vi "Get Device Parameters.vi"(8 "error in":errorcluster, 11 "custom device ref":T2=18446744073709551615 format="%.0x") -> (0 "error out":errorcluster, 2 "device parameters":T1, 3 "custom device ref out":T2 format="%.0x")   [LabVIEW 2020, in "AIM ARINC 429 Scripting.lvlib"]
doc: "Returns AIM hardware device parameters such as <b>pxi slot</b>."
uses:
  AIM ARINC 429 Scripting.lvlib
  <vilib>/NI VeriStand/Custom Device API/Custom Device Item Ref.ctl
  Shared/Device Parameters.ctl
  Constants.vi
  <vilib>/NI VeriStand/Custom Device API/Get Item Property (I32).vi
  <vilib>/NI VeriStand/Custom Device API/Custom Device API.lvlib
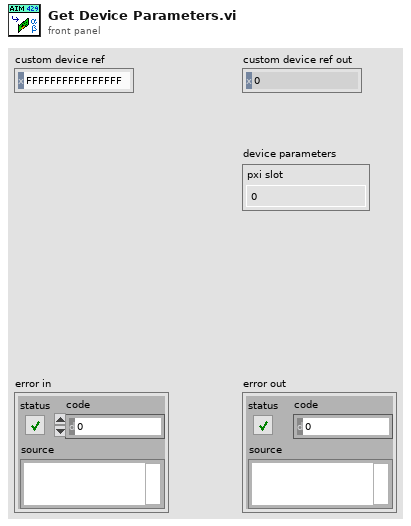
[diagram p1: front panel]
types:
  T1 = typedef "Device Parameters.ctl" = cluster{"pxi slot":u8}
  T2 = typedef "Custom Device API.lvlib/Custom Device Item Ref.ctl" = u64
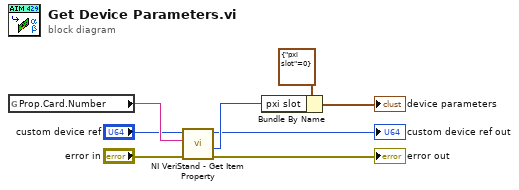
[diagram p0: block diagram]
diagram:
  n1 = global read "Constants.vi" "Prop.Card.Number"() -> (w7:string)
  n2 = call-poly <vilib>:"NI VeriStand - Get Item Property.vi"("error in (no error)"="error in", "Property Name"=w7, "Item Ref in"="custom device ref") -> ("error out"=→"error out":errorcluster, "Value"=w6:i32, "Item Ref out"=→"custom device ref out":T2)  [unwired: 5 in, 1 out]
  n3 = Bundle By Name(cluster=T1 {"pxi slot"=0} ("device parameters"), "pxi slot"=w6) -> (→"device parameters":T1)
